vi "CRYImport wizard top-level.vi"(10 "Data in flat (default empty)":string, 11 "Import path (just directory if no data input)":path=path "C:/SoundCheck 4.1/Data") -> (0 "Canceled?":bool, 2 "Data array out":string[](array[string]), 3 "Path out":path)   [LabVIEW 2013]
uses:
  Control/CRYImp wiz page flags.ctl
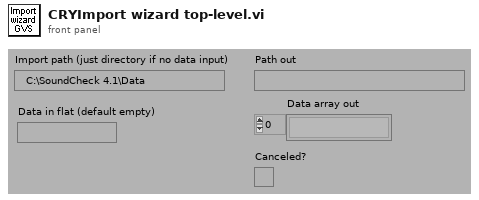
[diagram p1: front panel]
types:
  T1 = cluster{"import dir path":path, "datafile path":path, "file format":i32, "col delimiter":i32, "col other delim":string, "col width":i32, "rows/cols":i32, "offset cols":i32, "offset rows":i32, "header":bool, "header col":i32, "x axis layout":i32, "y axis layout":i32, "x start col":i32, "y start col":i32, "data incr":i32, "import settings path":path, "std hdr":bool}
  T2 = typedef "CRYImp wiz page flags.ctl" = cluster{"p1":bool, "p2":bool, "p3":bool, "p4":bool, "lb":bool, "finish":bool, "canceled":bool}
  T3 = typedef "CRYImp wiz main info.ctl" = cluster{"import dir path":path, "datafile path":path, "file format":i32, "col delimiter":i32, "col other delim":string, "col width":i32, "rows/cols":i32, "offset cols":i32, "offset rows":i32, "header":bool, "header col":i32, "x axis layout":i32, "y axis layout":i32, "x start col":i32, "y start col":i32, "data incr":i32, "import settings path":path, "std hdr":bool}
  T4 = typedef "CRYx-y settings array.ctl" = cluster{"x col":i32, "x data type":u16, "x axis type":u16, "x prefix":string, "x unit":string, "x db ref":dbl, "y col":i32, "Name:":string, "phase incl":bool, "ym data type":u16, "ym axis type":u16, "ym prefix":string, "ym unit":string, "ym db ref":dbl, "yp data type":u16, "yp axis type":u16, "yp prefix":string, "yp unit":string, "yp db ref":dbl}[]
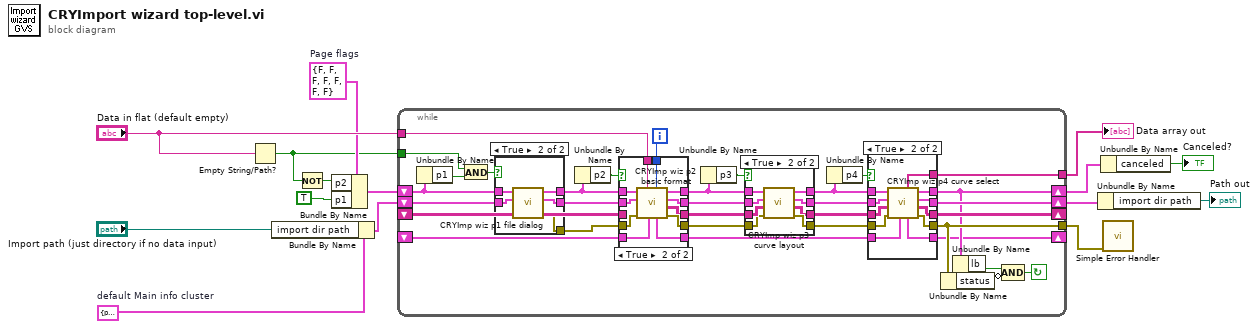
[diagram p0: block diagram]
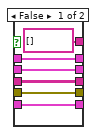
[diagram p3: hidden frame]
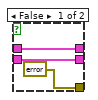
[diagram p5: hidden frame]
diagram:
  w13 = T1 {"import dir path"=path "", "datafile path"=path "", "file format"=0, "col delimiter"=0, "col other delim"="", "col width"=0, "rows/cols"=0, "offset cols"=0, "offset rows"=0, "header"=FALSE, "header col"=0, "x axis layout"=0, "y axis layout"=0, "x start col"=1, "y start col"=2, "data incr"=1, "import settings path"=path "", "std hdr"=FALSE}  # default Main info cluster
  w3 = T2 {"p1"=FALSE, "p2"=FALSE, "p3"=FALSE, "p4"=FALSE, "lb"=FALSE, "finish"=FALSE, "canceled"=FALSE}  # Page flags
  n1 = Empty String/Path?(string/path="Data in flat (default empty)") -> (empty?=w2:bool)
  n2 = Bundle By Name(cluster=w13, "import dir path"="Import path (just directory if no data input)") -> (w11:T1)
  n3 = Not(x=w2) -> (.not. x?=w1:bool)
  n4 = Bundle By Name(cluster=w3, "p2"=w1, "p1"=TRUE ("Bundle Element")) -> (w14:T2)
  n5 = while {
    tunnel: "Data in flat (default empty)" -> [w17]
    tunnel: w2 -> [w20]
    shift-left: _ -> [w22]
    shift-right: [w23] -> _
    tunnel: [w24] -> w5
    tunnel: [w30] -> w10
    shift-left: _ -> [w42]
    shift-right: [w29] -> _
    shift-left: w11 -> [w47]
    shift-right: [w28] -> w6
    shift-left: w14 -> [w48]
    shift-right: [w27] -> w8
    i -> [w16]
    stop <- w39 continue-if-true
    n6 = Unbundle By Name(w48) -> ("p1"=w19:bool)
    n7 = And(x=w20, y=w19) -> (x .and. y?=w18:bool)
    n8 = case shown="True" w18 {
      tunnel: w48 -> [w96 w101]
      tunnel: [w96 w98] -> w45
      tunnel: [w95 w99] -> w44
      tunnel: w47 -> [w95 w100]
      tunnel: [errorcluster {"status"=FALSE, "code"=0, "source"=""} ("error out") w97] -> w43
      frame False {
      }
      frame True {
        n9 = call "CRYImp wiz p1 file dialog.vi"("Main info cluster"=w100, "Page flags"=w101) -> ("error out"=w97:errorcluster, "Main info cluster out"=w99:T3, "Page flags out"=w98:T2)  [unwired: 7 in]
      }
    }
    n10 = Unbundle By Name(w45) -> ("p2"=w46:bool)
    n11 = case shown="True" w46 {
      tunnel: w45 -> [w82 w93]
      tunnel: [w82 w90] -> w37
      tunnel: [w81 w91] -> w36
      tunnel: w44 -> [w81 w92]
      tunnel: [w80 w89] -> w34
      tunnel: w43 -> [w80 w88]
      tunnel: [w79 w87] -> w35
      tunnel: w42 -> [w79 _]
      tunnel: w22 -> [w78 w86]
      tunnel: [w78 w85] -> w21
      tunnel: w17 -> [_ w84]
      tunnel: w16 -> [_ w83]
      frame False {
      }
      frame True {
        n12 = call "CRYImp wiz p2 basic format.vi"("Iteration"=w83, "x-y settings array"=w86, "Flat data in (optional)"=w84, "error in (no error)"=w88, "Main info cluster"=w92, "Page flags"=w93) -> ("error out"=w89:errorcluster, "Data out"=w87:string[][], "Main info cluster out"=w91:T3, "Page flags out"=w90:T2, "x-y settings array out"=w85:T4)  [unwired: 1 in]
      }
    }
    n13 = Unbundle By Name(w37) -> ("p3"=w38:bool)
    n14 = case shown="True" w38 {
      tunnel: w37 -> [w52 w60]
      tunnel: [w52 w53] -> w26
      tunnel: [w51 w54] -> w33
      tunnel: w36 -> [w51 w59]
      tunnel: [w50 w56] -> w31
      tunnel: w34 -> [w50 w57]
      tunnel: [w49 w55] -> w32
      tunnel: w35 -> [w49 w58]
      frame False {
      }
      frame True {
        n15 = call "CRYImp wiz p3 curve layout.vi"("error in (no error)"=w57, "Data in"=w58, "Main info cluster"=w59, "Page flags"=w60) -> ("error out"=w56:errorcluster, "Data out"=w55:string[][], "Main info cluster out"=w54:T3, "Page flags out"=w53:T2)  [unwired: 3 in, 1 out]
      }
    }
    n16 = Unbundle By Name(w26) -> ("p4"=w25:bool)
    n17 = case shown="True" w25 {
      tunnel: w26 -> [w66 w76]
      tunnel: [w66 w77] -> w27
      tunnel: [w65 w70] -> w28
      tunnel: w33 -> [w65 w75]
      tunnel: [w64 w72] -> w30
      tunnel: w31 -> [w64 w73]
      tunnel: [w63 w71] -> w29
      tunnel: w32 -> [w63 w74]
      tunnel: [string[] [] ("Data array out") w69] -> w24
      tunnel: [w61 w68] -> w23
      tunnel: w21 -> [w61 w67]
      frame False {
      }
      frame True {
        n18 = call "CRYImp wiz p4 curve select.vi"("x-y settings array"=w67, "error in (no error)"=w73, "Data in"=w74, "Main info cluster"=w75, "Page flags"=w76) -> ("error out"=w72:errorcluster, "Data out"=w71:string[][], "Main info cluster out"=w70:T3, "Page flags out"=w77:T2, "x-y settings array out"=w68:T4, "Data array out"=w69:string[])  [unwired: 1 in]
      }
    }
    n19 = Unbundle By Name(w30) -> ("status"=w41:bool)
    n20 = Unbundle By Name(w27) -> ("lb"=w40:bool)
    n21 = Compound Arithmetic op=AND(w40, invert w41) -> (w39:bool)
  }
  "Data array out" <- w5
  n22 = Unbundle By Name(w6) -> ("import dir path"=→"Path out":path)
  n23 = Unbundle By Name(w8) -> ("canceled"=→"Canceled?":bool)
  n24 = call <vilib>:"Simple Error Handler.vi"("error in (no error)"=w10) -> ()  [unwired: 1 in, 8 out]
